vi "SetTemp(SubVI).vi"(8 "error in (no error)":errorcluster, 10 "VISA resource name":refnum<visa-resource-name>="GPIB0::11::INSTR", 11 "Temp":dbl) -> (0 "error out":errorcluster, 2 "VISA resource name out":refnum<visa-resource-name>)   [LabVIEW 2020]
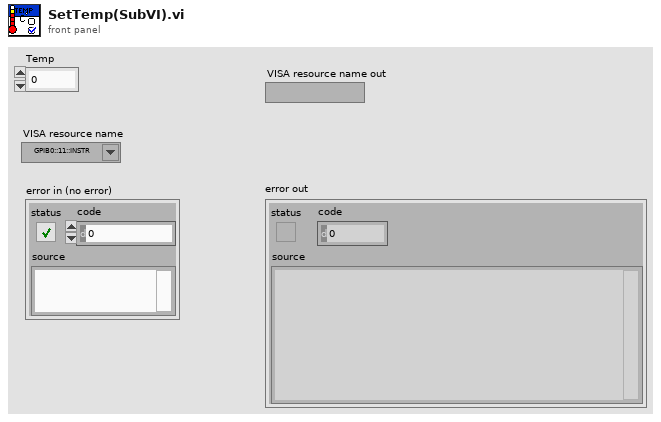
[diagram p1: front panel]
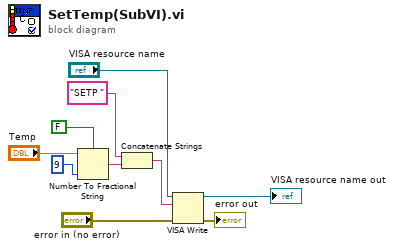
[diagram p0: block diagram]
diagram:
  n1 = Number To Fractional String(use system decimal point (T)=FALSE, number="Temp", precision (6)=i16 9) -> (F-format string=w7:string)  [unwired: 1 in]
  n2 = Concatenate Strings("SETP " ("write buffer"), w7) -> (w5:string)
  n3 = VISA Write(VISA resource name="VISA resource name", write buffer=w5, error in (no error)="error in (no error)") -> (VISA resource name out=→"VISA resource name out":refnum<visa-resource-name>, error out=→"error out":errorcluster)  [unwired: 1 out]
